vi "read_device_config.vi"() -> (0 "error out":errorcluster, 1 "device table":string[][](array[string]))   [LabVIEW 2026]
uses:
  <vilib>/addons/_office/excel.llb/Excel Get Data ([str]).vi
  <vilib>/Utility/NIReport.llb/NI_report.lvclass
  <vilib>/Utility/NIReport.llb/Excel/NI_Excel.lvclass
  <vilib>/addons/_office/NI_ReportGenerationToolkit.lvlib
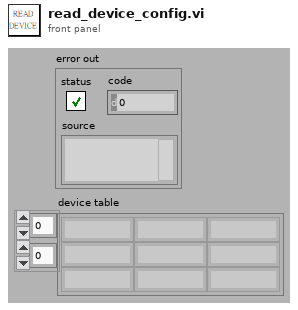
[diagram p1: front panel]
types:
  T1 = enum16{"maximized", "minimized", "normal", "no change"}
  T2 = enum16{"Standard Report", "HTML", "Word", "Excel"}
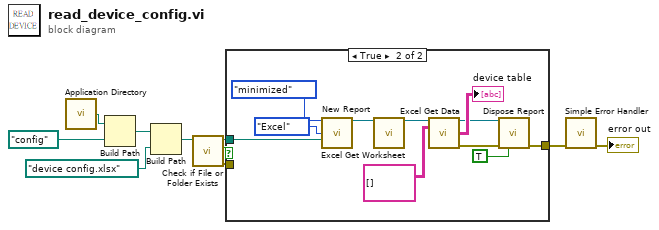
[diagram p0: block diagram]
diagram:
  n1 = call <vilib>:"Application Directory.vi"() -> ("Application Directory"=w10:path)
  n2 = Build Path(base path=w10, name or relative path=path "config") -> (appended path=w5:path)
  n3 = Build Path(base path=w5, name or relative path=path "device config.xlsx") -> (appended path=w4:path)
  n4 = call <vilib>:"Check if File or Folder Exists.vi"("path"=w4) -> ("error out"=w1:errorcluster, "file or folder exists?"=w3:bool, "dup path"=w2:path)  [unwired: 8 in]
  n5 = case shown="True" w3 {
    tunnel: [w11 w17] -> w6
    tunnel: w2 -> [_ w13]
    tunnel: w1 -> [w11 _]
    frame False {
    }
    frame True {
      n6 = call <vilib>:"New Report.vi"("window state (normal)"=T1."minimized", "report type"=T2."Excel", "template (empty)"=w13) -> ("report out"=w21:refnum<class "NI_report.lvclass">)  [unwired: 11 in, 1 out]
      n7 = call <vilib>:"Excel Get Worksheet.vi"("report in"=w21) -> ("report out"=w20:refnum<class "NI_report.lvclass">)  [unwired: 13 in, 1 out]
      n8 = call-poly <vilib>:"Excel Get Data.vi"("report in"=w20, "data type"=string[][] []) -> ("report out"=w15:refnum<class "NI_report.lvclass">, "data"=→"device table":string[][], "error out"=w14:errorcluster)  [unwired: 11 in]
      n9 = call-dynamic "Dispose Report.vi"("report in"=w15, "error in (no error)"=w14, "close report? (T)"=TRUE ("Close Report? (T)")) -> ("error out"=w17:errorcluster)  [unwired: 12 in]
    }
  }
  n10 = call <vilib>:"Simple Error Handler.vi"("error in (no error)"=w6) -> ("error out"=→"error out":errorcluster)  [unwired: 4 in, 4 out]
